vi "RampRate.vi"(8 "error in (no error)":errorcluster, 10 "Ramp rate (A/s)":dbl format="%#_13g", 11 "PS Driver AMI4xx in":refnum<class "PS Driver AMI4xx.lvclass">) -> (0 "error out":errorcluster, 2 "Ramp rate out (A/s)":dbl format="%#_13g", 3 "PS Driver AMI4xx out":refnum<class "PS Driver AMI4xx.lvclass">)   [LabVIEW 2019, in "PS Driver.lvlib" / "PS Driver AMI4xx.lvclass"]
uses:
  PS Driver AMI4xx.lvclass
  Y:/Winders Shared Folders/Interlock/SCM_PS_AF/PS Driver/PS Driver.lvclass
  PS Driver with Persistence.lvclass
  PS Driver.lvclass
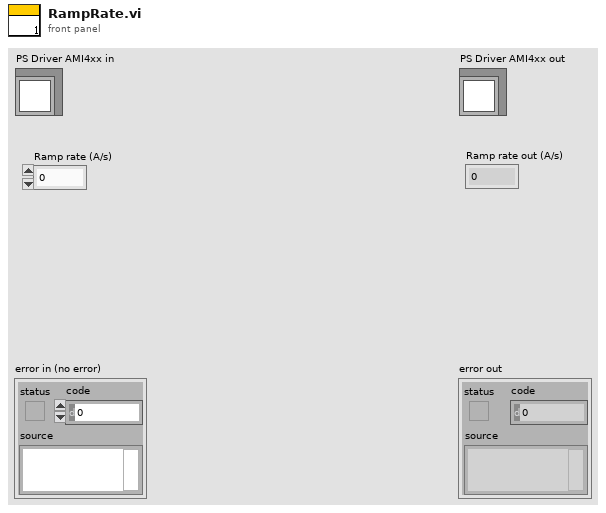
[diagram p1: front panel]
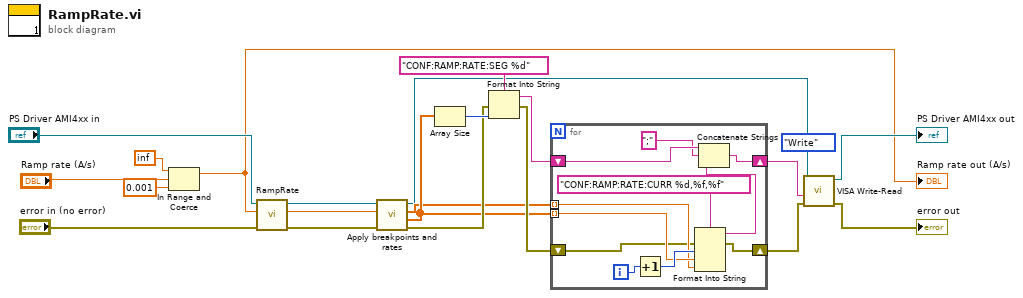
[diagram p0: block diagram]
diagram:
  n1 = In Range and Coerce(upper limit=inf, x="Ramp rate (A/s)", lower limit=0.001) -> (coerced(x)=w4:dbl)  [unwired: 1 out]
  "Ramp rate out (A/s)" <- w4
  n2 = call-parent "RampRate.vi"("error in (no error)"="error in (no error)", "Ramp rate (A/sec)"=w4, "PS Driver in"="PS Driver AMI4xx in") -> ("error out"=w20:errorcluster, "Ramp rate out (A/s)"=w19:dbl, "PS Driver out"=w18:refnum<class "PS Driver AMI4xx.lvclass">)  [unwired: 6 in]
  n3 = call "Apply breakpoints and rates.vi"("error in (no error)"=w20, "Ramp rate (A/sec)"=w19, "PS Driver in"=w18) -> ("error out"=w15:errorcluster, "Rates (A/sec)"=w12:dbl[], "Breakpoints (A)"=w11:dbl[], "PS Driver out"=w9:refnum<class "PS Driver AMI4xx.lvclass">)  [unwired: 5 in]
  n4 = Array Size(array=w12) -> (size(s)=w16:i32)
  n5 = Format Into String(format string="CONF:RAMP:RATE:SEG %d", error in=w15, w16) -> (resulting string=w13:string, error out=w14:errorcluster)  [unwired: 1 in]
  n6 = for {
    shift-right: [w26] -> w8
    shift-left: w14 -> [w28]
    shift-right: [w25] -> w10
    shift-left: w13 -> [w24]
    tunnel: w12 -> [w30] mode=indexing
    tunnel: w11 -> [w29] mode=indexing
    i -> [w33]
    n7 = Increment(x=w33) -> (x+1=w31:i32)
    n8 = Format Into String(format string="CONF:RAMP:RATE:CURR %d,%f,%f", error in=w28, w31, w30, w29) -> (resulting string=w27:string, error out=w26:errorcluster)  [unwired: 1 in]
    n9 = Concatenate Strings(w24, ";" ("string"), w27) -> (w25:string)
  }
  n10 = call "VISA Write-Read.vi"("error in (no error)"=w8, "Command String"=w10, "Action"=enum16{"Write", "Read", "Write & Read"}."Write", "PS Driver.lvlib:PS Driver AMI4xx.lvclass"=w9) -> ("error out"=→"error out":errorcluster, "PS Driver.lvlib:PS Driver AMI4xx.lvclass out"=→"PS Driver AMI4xx out":refnum<class "PS Driver AMI4xx.lvclass">)  [unwired: 4 in, 2 out]
